vi "Parse Table HTML SEARCHABLE.vi"(11 "array of devices":T1) -> (3 "String":string)   [LabVIEW 2016]
uses:
  Array Device Info.ctl
  Device Info.ctl
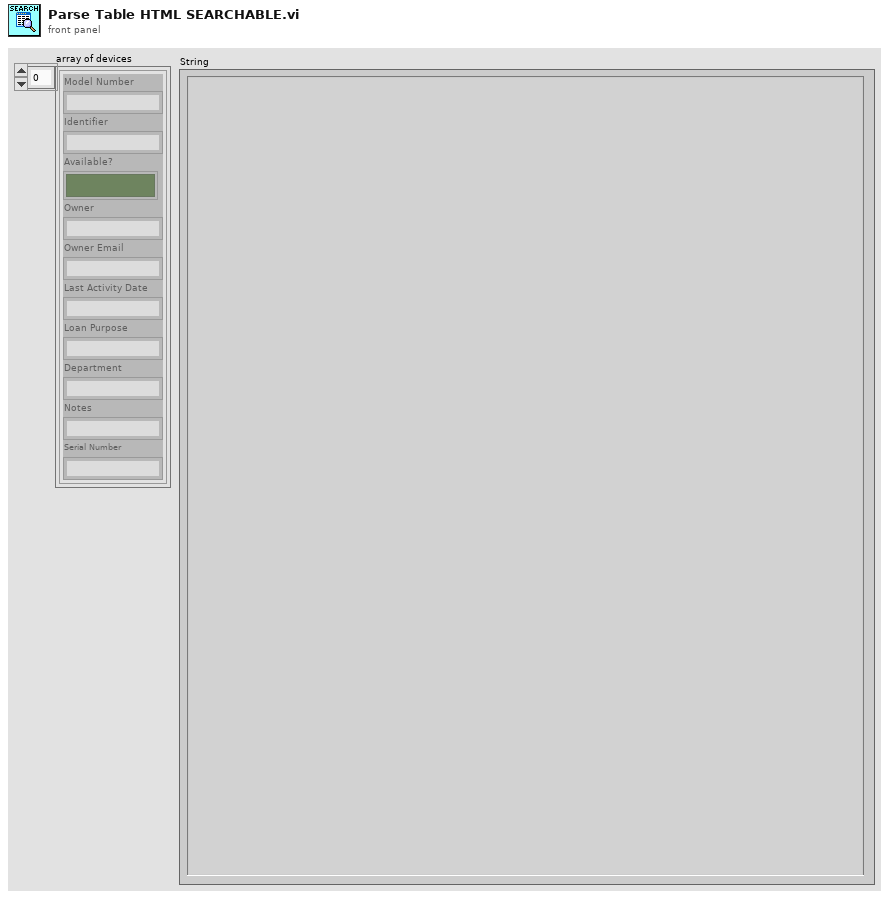
[diagram p1: front panel]
types:
  T1 = typedef "Array Device Info.ctl" = T2[]
  T2 = typedef "Device Info.ctl" = cluster{"Model Number":string, "Identifier":string, "Available?":bool, "Owner":string, "Owner Email":string, "Last Activity Date":string, "Loan Purpose":string, "Department":string, "Notes":string, "Serial Number":string}
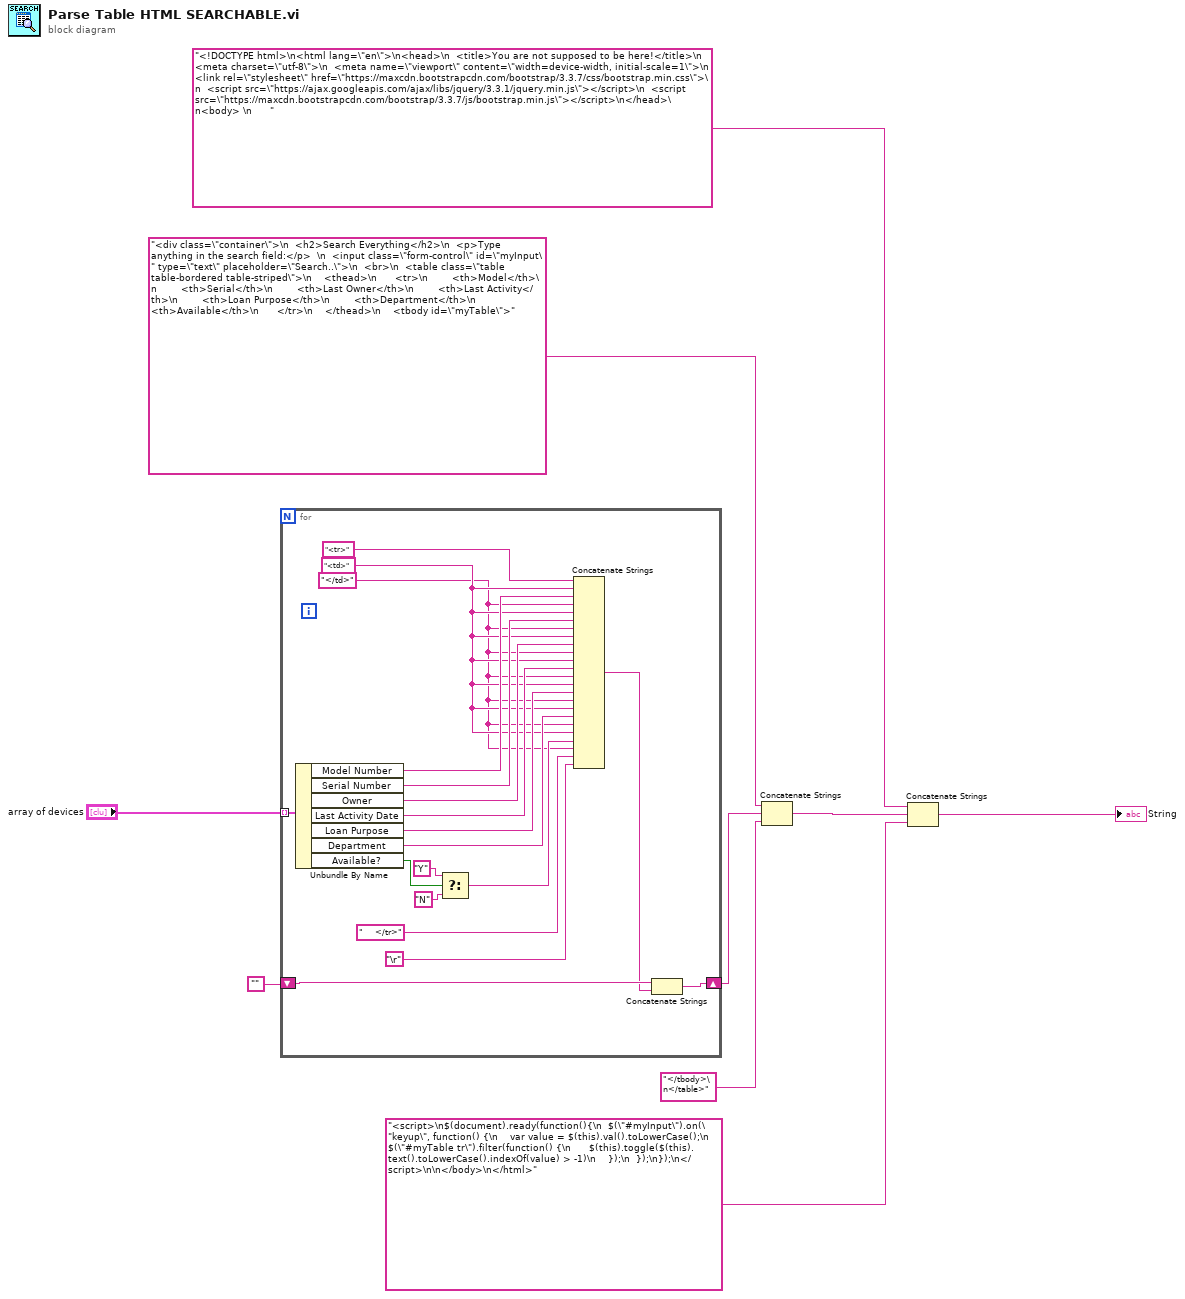
[diagram p0: block diagram]
diagram:
  n1 = for {
    tunnel: "array of devices" -> [w28] mode=indexing
    shift-right: [w26] -> w3
    shift-left: "" -> [w27]
    w14 = "<td>"
    w12 = "</td>"
    n2 = Unbundle By Name(w28) -> ("Model Number"=w25:string, "Serial Number"=w24:string, "Owner"=w23:string, "Last Activity Date"=w22:string, "Loan Purpose"=w21:string, "Department"=w20:string, "Available?"=w17:bool)
    n3 = Select(t="Y", s=w17, f="N") -> (s? t:f=w13:string)
    n4 = Concatenate Strings("<tr>", w14, w25, w12, w14, w24, w12, w14, w23, w12, w14, w22, w12, w14, w21, w12, w14, w20, w12, w14, w13, w12, "    </tr>", "\r") -> (w19:string)
    n5 = Concatenate Strings(w27, w19) -> (w26:string)
  }
  n6 = Concatenate Strings("<div class=\"container\">\n  <h2>Search Everything</h2>\n  <p>Type anything in the search field:</p>  \n  <input class=\"form-control\" id=\"myInput\" type=\"text\" placeholder=\"Search..\">\n  <br>\n  <table class=\"table table-bordered table-striped\">\n    <thead>\n      <tr>\n        <th>Model</th>\n        <th>Serial</th>\n        <th>Last Owner</th>\n        <th>Last Activity</th>\n        <th>Loan Purpose</th>\n        <th>Department</th>\n        <th>Available</th>\n      </tr>\n    </thead>\n    <tbody id=\"myTable\">", w3, "</tbody>\n</table>") -> (w7:string)
  n7 = Concatenate Strings("<!DOCTYPE html>\n<html lang=\"en\">\n<head>\n  <title>You are not supposed to be here!</title>\n  <meta charset=\"utf-8\">\n  <meta name=\"viewport\" content=\"width=device-width, initial-scale=1\">\n  <link rel=\"stylesheet\" href=\"https://maxcdn.bootstrapcdn.com/bootstrap/3.3.7/css/bootstrap.min.css\">\n  <script src=\"https://ajax.googleapis.com/ajax/libs/jquery/3.3.1/jquery.min.js\"></script>\n  <script src=\"https://maxcdn.bootstrapcdn.com/bootstrap/3.3.7/js/bootstrap.min.js\"></script>\n</head>\n<body> \n      ", w7, "<script>\n$(document).ready(function(){\n  $(\"#myInput\").on(\"keyup\", function() {\n    var value = $(this).val().toLowerCase();\n    $(\"#myTable tr\").filter(function() {\n      $(this).toggle($(this).text().toLowerCase().indexOf(value) > -1)\n    });\n  });\n});\n</script>\n\n</body>\n</html>") -> (→"String":string)
